vi "Set DAC.vi"(8 "error in (no error)":errorcluster, 9 "value (0)":i32, 10 "chan (0)":i32 min=0 max=1, 11 "VISA resource name":refnum<visa-resource-name>) -> (0 "error out":errorcluster, 3 "VISA resource name out":refnum<visa-resource-name>)   [LabVIEW 2025, in "Detector SCPI.lvlib"]
doc: "Sets voltage at DAC output\nChan is channel (0:1)\nVoltage is DAC output (0:4095)"
uses:
  Detector SCPI.lvlib
panel:
  out "Error Message":string
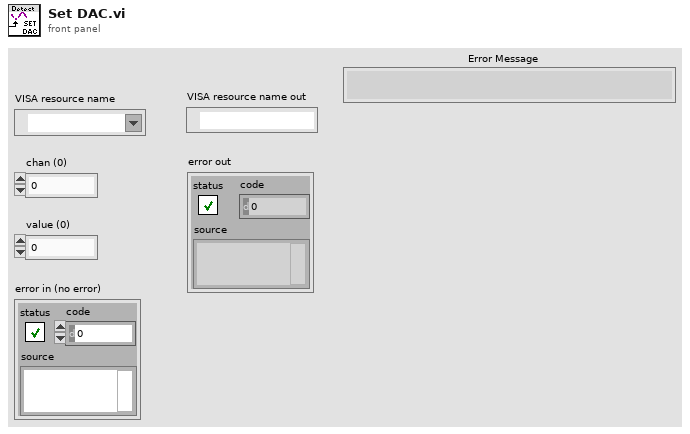
[diagram p1: front panel]
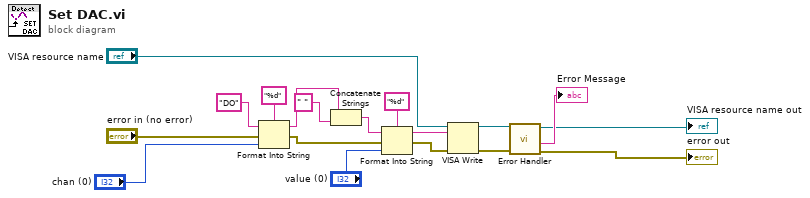
[diagram p0: block diagram]
diagram:
  n1 = Format Into String(format string="%d", initial string="DO" ("command"), error in="error in (no error)", "chan (0)") -> (resulting string=w10:string, error out=w16:errorcluster)
  n2 = Concatenate Strings(w10, " " ("command")) -> (w9:string)
  n3 = Format Into String(format string="%d", initial string=w9, error in=w16, "value (0)") -> (resulting string=w6:string, error out=w12:errorcluster)
  n4 = VISA Write(VISA resource name="VISA resource name", write buffer=w6, error in (no error)=w12) -> (VISA resource name out=w2:refnum<visa-resource-name>, error out=w4:errorcluster)  [unwired: 1 out]
  n5 = call "Error Handler.vi"("error in (no error)"=w4, "VISA resource name"=w2) -> ("error out"=→"error out":errorcluster, "Error Message"=→"Error Message":string, "VISA resource name out"=→"VISA resource name out":refnum<visa-resource-name>)  [unwired: 7 in]
